vi "Emballage_BDD_chargement_param_BLOCS_MEDIC.vi"(8 "Error in":errorcluster caption="Error in (no error)") -> (0 "Error out":errorcluster, 2 "Result Set":string[][](table) caption="Result Set (from first statement with results)", 3 "Column Names":string[](array[string]))   [LabVIEW 2020]
uses:
  Modules/FS/60_FS_Controles/60_FS_SetGet.ctl
  <vilib>/drjdpowell/SQLite Library/SQL Connection/Open (path).vi
  <vilib>/drjdpowell/SQLite Library/SQL Connection/Open (string).vi
  <vilib>/AdvancedString/Path To Command Line String.vi
  <vilib>/drjdpowell/SQLite Library/SQL Connection/Connection.lvclass
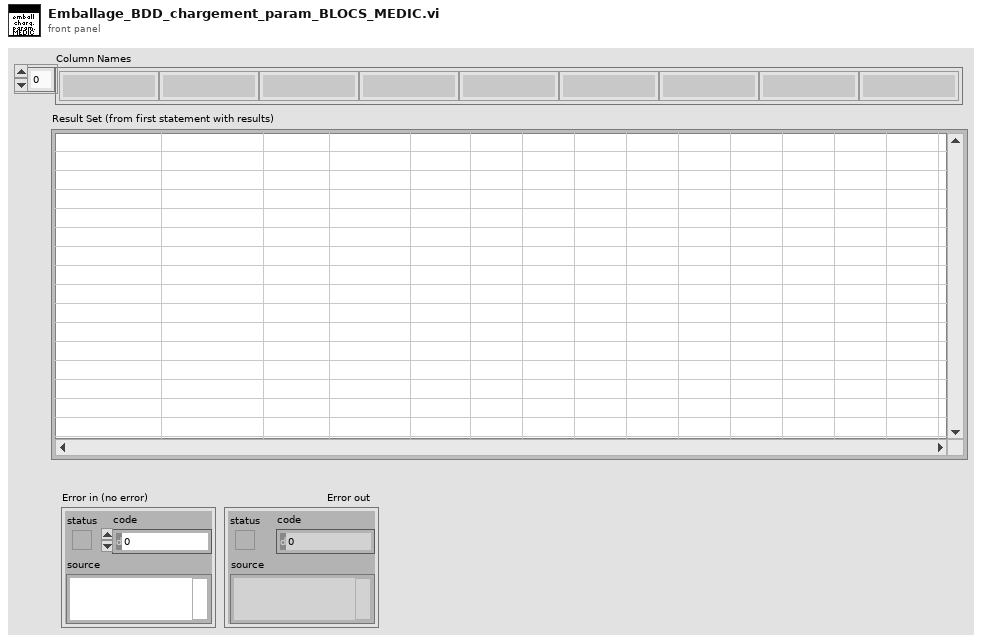
[diagram p1: front panel]
types:
  T1 = typedef "60_FS_SetGet.ctl" = enum16{"set", "get"}
  T2 = typedef "60_FS_CLT_Chemins.ctl" = cluster{"Racine_local":path, "Racine_reseau":path, "Racine_Support_Application":path, "Fichier_Journalisation":path, "Connexion_BDD_VSX":path, "Connexion_BDD_PLZ":path}
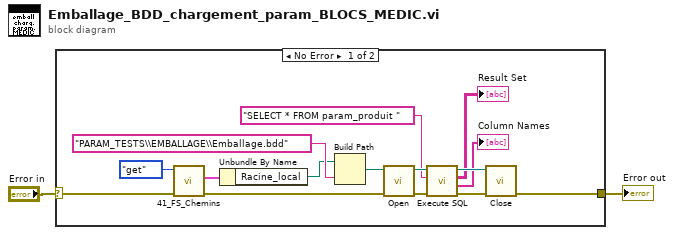
[diagram p0: block diagram]
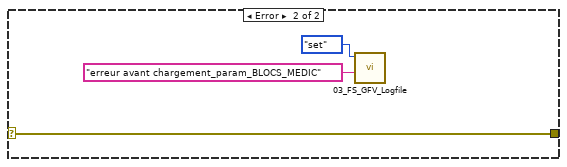
[diagram p2: hidden frame]
diagram:
  n1 = case shown="No Error" "Error in" {
    selector: "Error in" -> [w3 w20]
    tunnel: [w4 w20] -> w2
    frame No Error {
      n2 = call "41_FS_Chemins.vi"("error in (no error)"=w3, "SetGet"=60_FS_SetGet."get") -> ("error out"=w10:errorcluster, "CLT_Chemins_out"=w9:T2)  [unwired: 8 in]
      n3 = Unbundle By Name(w9) -> ("Racine_local"=w16:path)
      n4 = Build Path(base path=w16, name or relative path="PARAM_TESTS\\EMBALLAGE\\Emballage.bdd" ("nom ou chemin relatif")) -> (appended path=w15:path)
      n5 = call-poly <vilib>:"Open.vi"("error in (no error)"=w10, "db file"=w15) -> ("error out"=w6:errorcluster, "SQLite Connection"=w14:refnum<class "Connection.lvclass">)  [unwired: 8 in]
      n6 = call <vilib>:"Execute SQL.vi"("error in (no error)"=w6, "SQL"="SELECT * FROM param_produit ", "SQLite Connection in"=w14) -> ("error out"=w12:errorcluster, "Column Names"=→"Column Names":string[], "Result Set"=→"Result Set":string[][], "SQLite Connection"=w13:refnum<class "Connection.lvclass">)  [unwired: 5 in]
      n7 = call-dynamic "Close.vi"("error in (no error)"=w12, "SQLite Connection in"=w13) -> ("error out"=w4:errorcluster)  [unwired: 9 in]
    }
    frame Error {
      n8 = call "03_FS_GFV_Logfile.vi"("Chaîne"="erreur avant chargement_param_BLOCS_MEDIC", "States"=60_FS_SetGet."set") -> ()  [unwired: 8 in, 2 out]
    }
  }
  "Error out" <- w2
